vi "Password Authentication.vi"(8 "Error In":errorcluster, 9 "Password":string, 10 "Username":string, 11 "Session In":refnum<class "Session.lvclass">) -> (0 "Error Out":errorcluster, 3 "Sesssion Out":refnum<class "Session.lvclass">)   [LabVIEW 2017, in "Toolkit.lvlib" / "Session.lvclass"]
uses:
  Session.lvclass
  Session.lvclass/Session.ctl
  Toolkit.lvlib
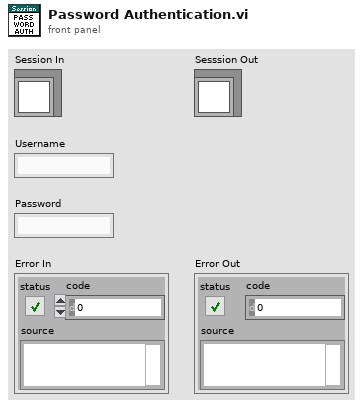
[diagram p1: front panel]
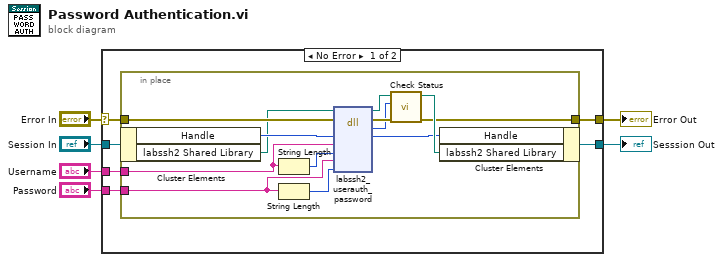
[diagram p0: block diagram]
diagram:
  n1 = case shown="No Error" "Error In" {
    selector: "Error In" -> [w9 w27]
    tunnel: [w11 w27] -> w5
    tunnel: "Session In" -> [w10 w26]
    tunnel: [w12 w26] -> w3
    tunnel: "Username" -> [w8 _]
    tunnel: "Password" -> [w7 _]
    frame No Error {
      n2 = in-place {
        in-place-border: [w22] -> w11
        in-place-border: w9 -> [w18]
        in-place-border: w8 -> [w16]
        in-place-border: w7 -> [w14]
        n3 = in-place-cluster #1(w10) -> ("Handle"=w21:u64, "labssh2 Shared Library"=w17:path)
        n4 = String Length(string=w16) -> (length=w15:i32)
        n5 = String Length(string=w14) -> (length=w13:i32)
        n6 = dll-call lib="D:/Users/cfield/Code/Field R&D Services/SSH/LabSSH2/LabVIEW/trunk/src/Toolkit/Support/labssh2.*" fn="labssh2_userauth_password"(path in=w17, error in=w18, "session"=w21, "username"=w16, "username_length"=w15, "password"=w14, "password_length"=w13) -> (path out=w25:path, error out=w23:errorcluster, "result"=w19:i32, "session"=w20:u64)  [unwired: 5 in]
        n7 = call "Check Status.vi"("Error In"=w23, "Status"=w19, "labssh2 Shared Library In"=w25) -> ("Error Out"=w22:errorcluster, "labssh2 Shared Library Out"=w24:path)  [unwired: 7 in]
        n8 = in-place-cluster #1("Handle"=w20, "labssh2 Shared Library"=w24) -> (w12:refnum<class "Session.lvclass">)
      }
    }
    frame Error {
    }
  }
  "Sesssion Out" <- w3
  "Error Out" <- w5
